vi "VG_TusineMax.vi"() -> ()   [LabVIEW 2020]
panel:
  out "TusineMax":dbl
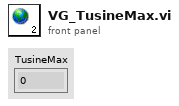
[diagram p1: front panel]
diagram:
